vi "Browse.vi"(4 "pathnameIN":path caption="Path Name", 7 "filename":string="file name" caption="File Name") -> (0 "pathname":path caption="Path Name", 1 "canceled":bool caption="Canceled", 2 "exists":bool caption="Exists", 3 "filenameOUT":string caption="File Name")   [LabVIEW 2017]
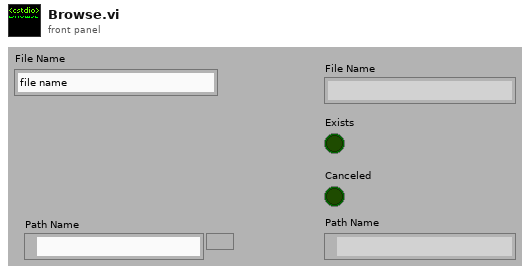
[diagram p1: front panel]
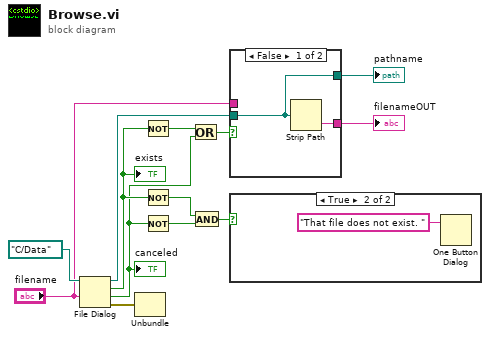
[diagram p0: block diagram]
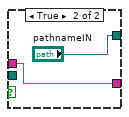
[diagram p3: hidden frame]
diagram:
  n1 = File Dialog(9:"filename", 11:path "C:/Data") -> (0:w1:errorcluster, 1:w2:bool, 2:w3:bool, 3:w9:path)  [unwired: 1 in, 4 out]
  "exists" <- w3
  "canceled" <- w2
  n2 = Unbundle(w1) -> ()  [unwired: 3 out]
  n3 = Not(x=w3) -> (.not. x?=w10:bool)
  n4 = Not(x=w3) -> (.not. x?=w4:bool)
  n5 = Not(x=w2) -> (.not. x?=w5:bool)
  n6 = Or(x=w10, y=w2) -> (x .or. y?=w11:bool)
  n7 = And(x=w4, y=w5) -> (x .and. y?=w6:bool)
  n8 = case shown="False" w11 {
    tunnel: w9 -> [w15 _]
    tunnel: [w14 w17] -> w12
    tunnel: "filename" -> [_ w17]
    tunnel: [w15 "pathnameIN"] -> w7
    frame False {
      n9 = Strip Path(path=w15) -> (name=w14:string)  [unwired: 1 out]
    }
    frame True {
    }
  }
  "pathname" <- w7
  "filenameOUT" <- w12
  n10 = case shown="True" w6 {
    frame False {
    }
    frame True {
      n11 = One Button Dialog(message="That file does not exist. ") -> ()  [unwired: 2 out]
    }
  }
